vi "Create Command Packet 3.vi"(0 "CCD Format Parameters":T1={"Serial Origin"=50, "Serial Length"=512, "Serial Binning"=1, "Parallel Origin"=0, "Parallel Length"=1024, "Parallel Binning"=1} {"Parallel Binning" min=1 max=5000 step=1; "Parallel Length" min=0 max=65535 step=1; "Parallel Origin" min=0 max=9000 step=1; "Serial Binning" min=1 max=5000 step=1; "Serial Length" min=0 max=65535 step=1; "Serial Origin" min=0 max=9000 step=1}, 4 "Save As":u16(ring) items=["U16 FITS", "I16 FITS", "I32 FITS", "SGL FITS", "U16 TIFF", "I16 TIFF", "I32 TIFF", "SGL TIFF"], 5 "Acq. Mode/Type/Frame Mode/RO Mode":u8, 6 "File Name":string, 7 "Camera ID (1)":u8=1, 8 "Mode":u16, 9 "Exposure Time (ms)":u32, 10 "Buffer/Avg #/Frames":u16, 11 "Function #":u16) -> (2 "Cmd Packet":string)   [LabVIEW 2015]
uses:
  CCD Format.ctl
panel:
  # "Parallel"
  # "Serial"
  # "Origin"
  # "Length"
  # "Binning"
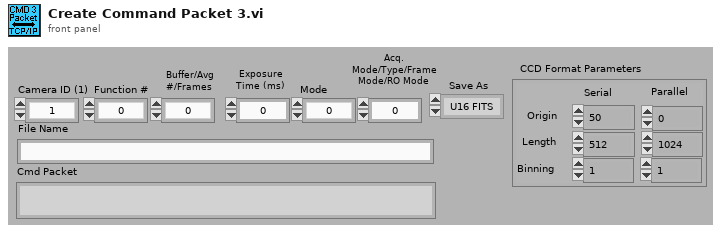
[diagram p1: front panel]
types:
  T1 = typedef "CCD Format.ctl" = cluster{"Serial Origin":i32, "Serial Length":i32, "Serial Binning":i32, "Parallel Origin":i32, "Parallel Length":i32, "Parallel Binning":i32}
  T2 = cluster{"Packet Length":u32, u8, "Camera ID (1)":u8, "Function #":u16, "Param Block Length":u16}
  T3 = cluster{u32, u8, "Camera ID (1)":u8, "Function #":u16, u16, "Exposure Time (ms)":u32, "Mode":u16, "Buffer/Avg #/Frames":u16, "Save As":u16}
  T4 = cluster{"Packet Length":u32, u8, "Camera ID (1)":u8, "Function #":u16, "Param Block Length":u16, "Buffer/Avg #/Frames":u16}
  T5 = cluster{u32, u8, "Camera ID (1)":u8, "Function #":u16, u16, "Buffer/Avg #/Frames":u16, "Save As":u16}
  T6 = cluster{"Packet Length":u32, u8, "Camera ID (1)":u8, "Function #":u16, "Param Block Length":u16, "Acq. Mode/Type/Frame Mode/RO Mode":u8}
  T7 = cluster{"Packet Length":u32, u8, "Camera ID (1)":u8, "Function #":u16, "Param Block Length":u16, "Exposure Time (ms)":u32}
  T8 = cluster{"Packet Length":u32, u8, "Camera ID (1)":u8, "Function #":u16, "Param Block Length":u16, "Buffer/Avg #/Frames":u16, "Acq. Mode/Type/Frame Mode/RO Mode":u8}
  T9 = cluster{u32, u8, "Camera ID (1)":u8, "Function #":u16, u16, "Mode":u16, "Buffer/Avg #/Frames":u16, "Save As":u16}
  T10 = cluster{"Packet Length":u32, u8, "Camera ID (1)":u8, "Function #":u16, "Param Block Length":u16, "CCD Format Parameters":T1}
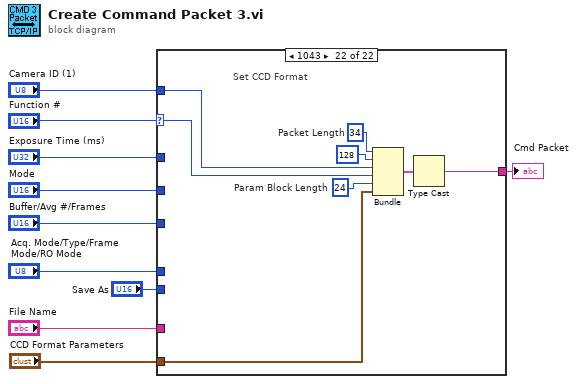
[diagram p0: block diagram]
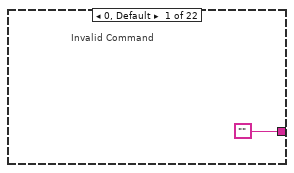
[diagram p2: hidden frame]
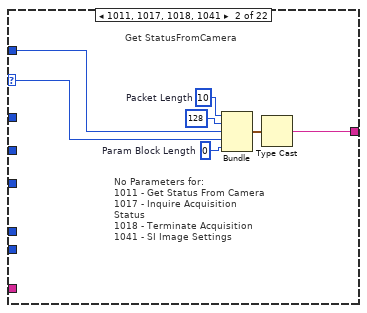
[diagram p3: hidden frame]
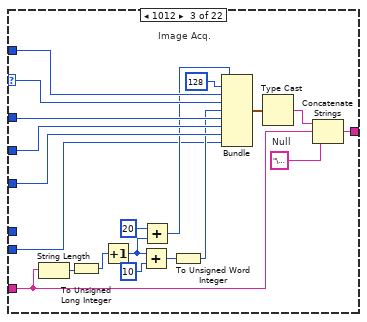
[diagram p4: hidden frame]
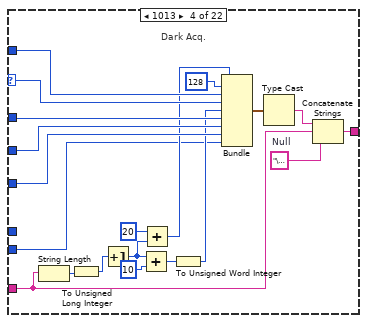
[diagram p5: hidden frame]
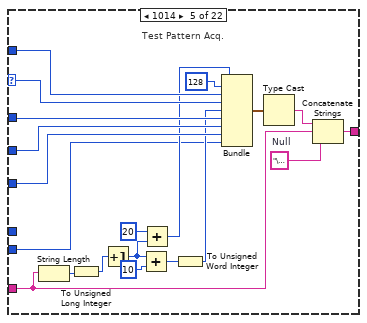
[diagram p6: hidden frame]
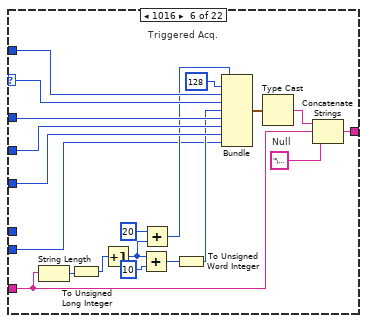
[diagram p7: hidden frame]
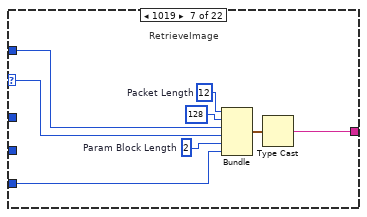
[diagram p8: hidden frame]
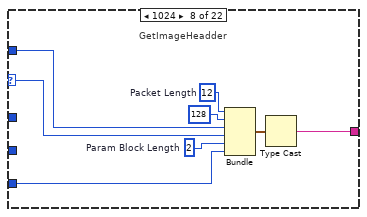
[diagram p9: hidden frame]
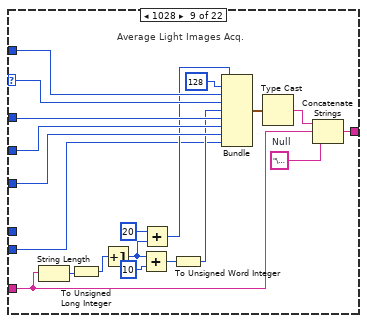
[diagram p10: hidden frame]
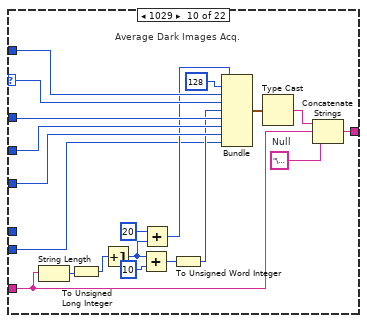
[diagram p11: hidden frame]
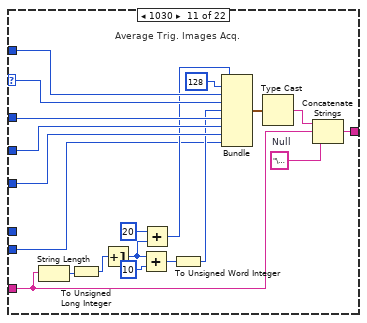
[diagram p12: hidden frame]
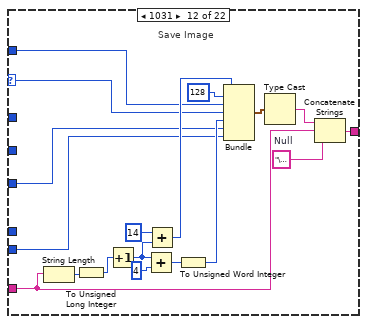
[diagram p13: hidden frame]
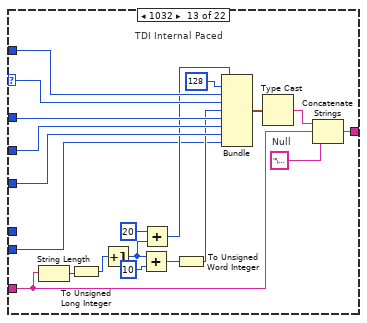
[diagram p14: hidden frame]
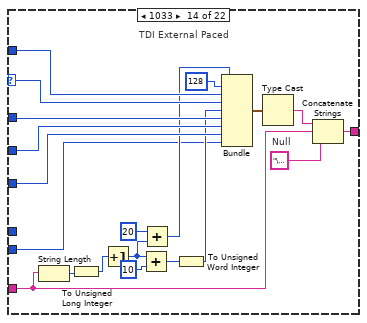
[diagram p15: hidden frame]
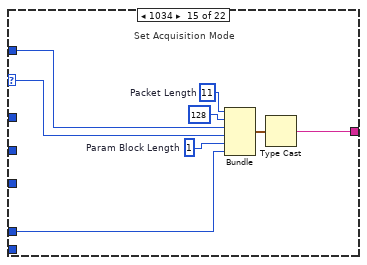
[diagram p16: hidden frame]
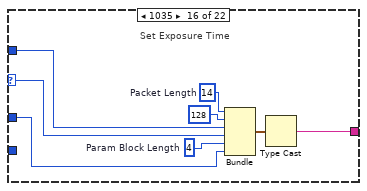
[diagram p17: hidden frame]
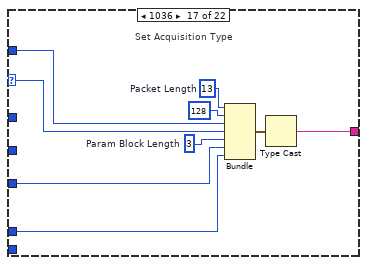
[diagram p18: hidden frame]
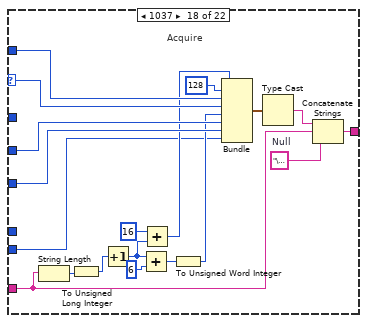
[diagram p19: hidden frame]
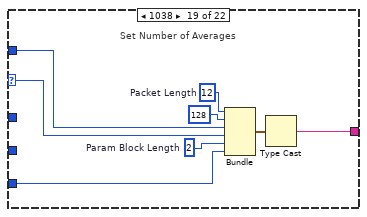
[diagram p20: hidden frame]
diagram:
  n1 = case shown="1043" "Function #" {
    selector: "Function #" -> [_ w15 w35 w55 w75 w95 w103 w109 w131 w151 w171 w176 w209 w229 w235 w243 w252 w273 w279 w287 w295 w303]
    tunnel: "Camera ID (1)" -> [_ w16 w36 w56 w76 w96 w104 w110 w132 w152 w172 w175 w210 w230 w236 w244 w253 w274 w280 w288 w296 w304]
    tunnel: "Exposure Time (ms)" -> [_ _ w34 w54 w74 w94 _ _ w130 w150 w170 _ w208 w228 _ w241 _ _ _ _ _ _]
    tunnel: "Mode" -> [_ _ w33 w53 w73 w93 _ _ w129 w149 w169 _ w207 w227 _ _ _ w272 _ _ _ _]
    tunnel: "Buffer/Avg #/Frames" -> [_ _ w32 w52 w72 w92 w102 w108 w128 w148 w168 w178 w206 w226 _ _ w249 w271 w277 w285 _ _]
    tunnel: "File Name" -> [_ _ w23 w43 w63 w83 _ _ w119 w139 w159 w180 w197 w217 _ _ _ w262 _ _ _ _]
    tunnel: ["" w12 w21 w41 w61 w81 w99 w107 w117 w137 w157 w177 w195 w215 w234 w242 w251 w260 w278 w286 w294 w302] -> w4
    tunnel: "Save As" -> [_ _ w19 w39 w59 w79 _ _ w115 w135 w155 w179 w193 w213 _ _ _ w258 _ _ _ _]
    tunnel: "Acq. Mode/Type/Frame Mode/RO Mode" -> [_ _ _ _ _ _ _ _ _ _ _ _ _ _ w233 _ w250 _ _ _ w293 _]
    tunnel: "CCD Format Parameters" -> [_ _ _ _ _ _ _ _ _ _ _ _ _ _ _ _ _ _ _ _ _ w301]
    frame 0, Default {
      # "Invalid Command"
    }
    frame 1011, 1017, 1018, 1041 {
      w13 = u16 0  # Param Block Length
      w14 = u32 10  # Packet Length
      # "No Parameters for:\n1011 - Get Status From Camera\n1017 - Inquire Acquisition Status\n1018 - Terminate Acquisition\n1041 - SI Image Settings"
      # "Get StatusFromCamera"
      n2 = Bundle("Packet Length"=w14, u8 128, "Camera ID (1)"=w16, "Function #"=w15, "Param Block Length"=w13) -> (w17:T2)  [unwired: 1 in]
      n3 = Type Cast(x=w17) -> (*(type *) &x=w12:string)  [unwired: 1 in]
    }
    frame 1012 {
      w22 = "\u0000"  # Null
      # "Image Acq."
      n4 = String Length(string=w23) -> (length=w31:i32)
      n5 = To Unsigned Long Integer(number=w31) -> (unsigned 32bit integer=w29:u32)
      n6 = Increment(x=w29) -> (x+1=w30:u32)
      n7 = Add(x=w30, y=u16 10) -> (x+y=w25:u32)
      n8 = Add(x=u16 20, y=w30) -> (x+y=w26:u32)
      n9 = To Unsigned Word Integer(number=w25) -> (unsigned 16bit integer=w20:u16)
      n10 = Bundle(w26, u8 128, "Camera ID (1)"=w36, "Function #"=w35, w20, "Exposure Time (ms)"=w34, "Mode"=w33, "Buffer/Avg #/Frames"=w32, "Save As"=w19) -> (w37:T3)  [unwired: 1 in]
      n11 = Type Cast(x=w37) -> (*(type *) &x=w24:string)  [unwired: 1 in]
      n12 = Concatenate Strings(w24, w23, w22) -> (w21:string)
    }
    frame 1013 {
      w42 = "\u0000"  # Null
      # "Dark Acq."
      n13 = String Length(string=w43) -> (length=w51:i32)
      n14 = To Unsigned Long Integer(number=w51) -> (unsigned 32bit integer=w49:u32)
      n15 = Increment(x=w49) -> (x+1=w50:u32)
      n16 = Add(x=w50, y=u16 10) -> (x+y=w45:u32)
      n17 = Add(x=u16 20, y=w50) -> (x+y=w46:u32)
      n18 = To Unsigned Word Integer(number=w45) -> (unsigned 16bit integer=w40:u16)
      n19 = Bundle(w46, u8 128, "Camera ID (1)"=w56, "Function #"=w55, w40, "Exposure Time (ms)"=w54, "Mode"=w53, "Buffer/Avg #/Frames"=w52, "Save As"=w39) -> (w57:T3)  [unwired: 1 in]
      n20 = Type Cast(x=w57) -> (*(type *) &x=w44:string)  [unwired: 1 in]
      n21 = Concatenate Strings(w44, w43, w42) -> (w41:string)
    }
    frame 1014 {
      w62 = "\u0000"  # Null
      # "Test Pattern Acq."
      n22 = String Length(string=w63) -> (length=w71:i32)
      n23 = To Unsigned Long Integer(number=w71) -> (unsigned 32bit integer=w69:u32)
      n24 = Increment(x=w69) -> (x+1=w70:u32)
      n25 = Add(x=w70, y=u16 10) -> (x+y=w65:u32)
      n26 = Add(x=u16 20, y=w70) -> (x+y=w66:u32)
      n27 = To Unsigned Word Integer(number=w65) -> (unsigned 16bit integer=w60:u16)
      n28 = Bundle(w66, u8 128, "Camera ID (1)"=w76, "Function #"=w75, w60, "Exposure Time (ms)"=w74, "Mode"=w73, "Buffer/Avg #/Frames"=w72, "Save As"=w59) -> (w77:T3)  [unwired: 1 in]
      n29 = Type Cast(x=w77) -> (*(type *) &x=w64:string)  [unwired: 1 in]
      n30 = Concatenate Strings(w64, w63, w62) -> (w61:string)
    }
    frame 1016 {
      w82 = "\u0000"  # Null
      # "Triggered Acq."
      n31 = String Length(string=w83) -> (length=w91:i32)
      n32 = To Unsigned Long Integer(number=w91) -> (unsigned 32bit integer=w89:u32)
      n33 = Increment(x=w89) -> (x+1=w90:u32)
      n34 = Add(x=w90, y=u16 10) -> (x+y=w85:u32)
      n35 = Add(x=u16 20, y=w90) -> (x+y=w86:u32)
      n36 = To Unsigned Word Integer(number=w85) -> (unsigned 16bit integer=w80:u16)
      n37 = Bundle(w86, u8 128, "Camera ID (1)"=w96, "Function #"=w95, w80, "Exposure Time (ms)"=w94, "Mode"=w93, "Buffer/Avg #/Frames"=w92, "Save As"=w79) -> (w97:T3)  [unwired: 1 in]
      n38 = Type Cast(x=w97) -> (*(type *) &x=w84:string)  [unwired: 1 in]
      n39 = Concatenate Strings(w84, w83, w82) -> (w81:string)
    }
    frame 1019 {
      w100 = u16 2  # Param Block Length
      w101 = u32 12  # Packet Length
      # "RetrieveImage"
      n40 = Bundle("Packet Length"=w101, u8 128, "Camera ID (1)"=w104, "Function #"=w103, "Param Block Length"=w100, "Buffer/Avg #/Frames"=w102) -> (w105:T4)  [unwired: 1 in]
      n41 = Type Cast(x=w105) -> (*(type *) &x=w99:string)  [unwired: 1 in]
    }
    frame 1024 {
      w111 = u16 2  # Param Block Length
      w112 = u32 12  # Packet Length
      # "GetImageHeadder"
      n42 = Bundle("Packet Length"=w112, u8 128, "Camera ID (1)"=w110, "Function #"=w109, "Param Block Length"=w111, "Buffer/Avg #/Frames"=w108) -> (w113:T4)  [unwired: 1 in]
      n43 = Type Cast(x=w113) -> (*(type *) &x=w107:string)  [unwired: 1 in]
    }
    frame 1028 {
      w118 = "\u0000"  # Null
      # "Average Light Images Acq."
      n44 = String Length(string=w119) -> (length=w127:i32)
      n45 = To Unsigned Long Integer(number=w127) -> (unsigned 32bit integer=w125:u32)
      n46 = Increment(x=w125) -> (x+1=w126:u32)
      n47 = Add(x=w126, y=u16 10) -> (x+y=w121:u32)
      n48 = Add(x=u16 20, y=w126) -> (x+y=w122:u32)
      n49 = To Unsigned Word Integer(number=w121) -> (unsigned 16bit integer=w116:u16)
      n50 = Bundle(w122, u8 128, "Camera ID (1)"=w132, "Function #"=w131, w116, "Exposure Time (ms)"=w130, "Mode"=w129, "Buffer/Avg #/Frames"=w128, "Save As"=w115) -> (w133:T3)  [unwired: 1 in]
      n51 = Type Cast(x=w133) -> (*(type *) &x=w120:string)  [unwired: 1 in]
      n52 = Concatenate Strings(w120, w119, w118) -> (w117:string)
    }
    frame 1029 {
      w138 = "\u0000"  # Null
      # "Average Dark Images Acq."
      n53 = String Length(string=w139) -> (length=w147:i32)
      n54 = To Unsigned Long Integer(number=w147) -> (unsigned 32bit integer=w145:u32)
      n55 = Increment(x=w145) -> (x+1=w146:u32)
      n56 = Add(x=w146, y=u16 10) -> (x+y=w141:u32)
      n57 = Add(x=u16 20, y=w146) -> (x+y=w142:u32)
      n58 = To Unsigned Word Integer(number=w141) -> (unsigned 16bit integer=w136:u16)
      n59 = Bundle(w142, u8 128, "Camera ID (1)"=w152, "Function #"=w151, w136, "Exposure Time (ms)"=w150, "Mode"=w149, "Buffer/Avg #/Frames"=w148, "Save As"=w135) -> (w153:T3)  [unwired: 1 in]
      n60 = Type Cast(x=w153) -> (*(type *) &x=w140:string)  [unwired: 1 in]
      n61 = Concatenate Strings(w140, w139, w138) -> (w137:string)
    }
    frame 1030 {
      w158 = "\u0000"  # Null
      # "Average Trig. Images Acq."
      n62 = String Length(string=w159) -> (length=w167:i32)
      n63 = To Unsigned Long Integer(number=w167) -> (unsigned 32bit integer=w165:u32)
      n64 = Increment(x=w165) -> (x+1=w166:u32)
      n65 = Add(x=w166, y=u16 10) -> (x+y=w161:u32)
      n66 = Add(x=u16 20, y=w166) -> (x+y=w162:u32)
      n67 = To Unsigned Word Integer(number=w161) -> (unsigned 16bit integer=w156:u16)
      n68 = Bundle(w162, u8 128, "Camera ID (1)"=w172, "Function #"=w171, w156, "Exposure Time (ms)"=w170, "Mode"=w169, "Buffer/Avg #/Frames"=w168, "Save As"=w155) -> (w173:T3)  [unwired: 1 in]
      n69 = Type Cast(x=w173) -> (*(type *) &x=w160:string)  [unwired: 1 in]
      n70 = Concatenate Strings(w160, w159, w158) -> (w157:string)
    }
    frame 1031 {
      w182 = "\u0000"  # Null
      # "Save Image"
      n71 = String Length(string=w180) -> (length=w190:i32)
      n72 = To Unsigned Long Integer(number=w190) -> (unsigned 32bit integer=w188:u32)
      n73 = Increment(x=w188) -> (x+1=w189:u32)
      n74 = Add(x=w189, y=u16 4) -> (x+y=w184:u32)
      n75 = Add(x=u16 14, y=w189) -> (x+y=w185:u32)
      n76 = To Unsigned Word Integer(number=w184) -> (unsigned 16bit integer=w181:u16)
      n77 = Bundle(w185, u8 128, "Camera ID (1)"=w175, "Function #"=w176, w181, "Buffer/Avg #/Frames"=w178, "Save As"=w179) -> (w191:T5)  [unwired: 1 in]
      n78 = Type Cast(x=w191) -> (*(type *) &x=w183:string)  [unwired: 1 in]
      n79 = Concatenate Strings(w183, w180, w182) -> (w177:string)
    }
    frame 1032 {
      w196 = "\u0000"  # Null
      # "TDI Internal Paced"
      n80 = String Length(string=w197) -> (length=w205:i32)
      n81 = To Unsigned Long Integer(number=w205) -> (unsigned 32bit integer=w203:u32)
      n82 = Increment(x=w203) -> (x+1=w204:u32)
      n83 = Add(x=w204, y=u16 10) -> (x+y=w199:u32)
      n84 = Add(x=u16 20, y=w204) -> (x+y=w200:u32)
      n85 = To Unsigned Word Integer(number=w199) -> (unsigned 16bit integer=w194:u16)
      n86 = Bundle(w200, u8 128, "Camera ID (1)"=w210, "Function #"=w209, w194, "Exposure Time (ms)"=w208, "Mode"=w207, "Buffer/Avg #/Frames"=w206, "Save As"=w193) -> (w211:T3)  [unwired: 1 in]
      n87 = Type Cast(x=w211) -> (*(type *) &x=w198:string)  [unwired: 1 in]
      n88 = Concatenate Strings(w198, w197, w196) -> (w195:string)
    }
    frame 1033 {
      w216 = "\u0000"  # Null
      # "TDI External Paced"
      n89 = String Length(string=w217) -> (length=w225:i32)
      n90 = To Unsigned Long Integer(number=w225) -> (unsigned 32bit integer=w223:u32)
      n91 = Increment(x=w223) -> (x+1=w224:u32)
      n92 = Add(x=w224, y=u16 10) -> (x+y=w219:u32)
      n93 = Add(x=u16 20, y=w224) -> (x+y=w220:u32)
      n94 = To Unsigned Word Integer(number=w219) -> (unsigned 16bit integer=w214:u16)
      n95 = Bundle(w220, u8 128, "Camera ID (1)"=w230, "Function #"=w229, w214, "Exposure Time (ms)"=w228, "Mode"=w227, "Buffer/Avg #/Frames"=w226, "Save As"=w213) -> (w231:T3)  [unwired: 1 in]
      n96 = Type Cast(x=w231) -> (*(type *) &x=w218:string)  [unwired: 1 in]
      n97 = Concatenate Strings(w218, w217, w216) -> (w215:string)
    }
    frame 1034 {
      w237 = u16 1  # Param Block Length
      w238 = u32 11  # Packet Length
      # "Set Acquisition Mode"
      n98 = Bundle("Packet Length"=w238, u8 128, "Camera ID (1)"=w236, "Function #"=w235, "Param Block Length"=w237, "Acq. Mode/Type/Frame Mode/RO Mode"=w233) -> (w239:T6)  [unwired: 1 in]
      n99 = Type Cast(x=w239) -> (*(type *) &x=w234:string)  [unwired: 1 in]
    }
    frame 1035 {
      w245 = u16 4  # Param Block Length
      w246 = u32 14  # Packet Length
      # "Set Exposure Time"
      n100 = Bundle("Packet Length"=w246, u8 128, "Camera ID (1)"=w244, "Function #"=w243, "Param Block Length"=w245, "Exposure Time (ms)"=w241) -> (w247:T7)  [unwired: 1 in]
      n101 = Type Cast(x=w247) -> (*(type *) &x=w242:string)  [unwired: 1 in]
    }
    frame 1036 {
      w254 = u16 3  # Param Block Length
      w255 = u32 13  # Packet Length
      # "Set Acquisition Type"
      n102 = Bundle("Packet Length"=w255, u8 128, "Camera ID (1)"=w253, "Function #"=w252, "Param Block Length"=w254, "Buffer/Avg #/Frames"=w249, "Acq. Mode/Type/Frame Mode/RO Mode"=w250) -> (w256:T8)  [unwired: 1 in]
      n103 = Type Cast(x=w256) -> (*(type *) &x=w251:string)  [unwired: 1 in]
    }
    frame 1037 {
      w261 = "\u0000"  # Null
      # "Acquire"
      n104 = String Length(string=w262) -> (length=w270:i32)
      n105 = To Unsigned Long Integer(number=w270) -> (unsigned 32bit integer=w268:u32)
      n106 = Increment(x=w268) -> (x+1=w269:u32)
      n107 = Add(x=w269, y=u16 6) -> (x+y=w264:u32)
      n108 = Add(x=u16 16, y=w269) -> (x+y=w265:u32)
      n109 = To Unsigned Word Integer(number=w264) -> (unsigned 16bit integer=w259:u16)
      n110 = Bundle(w265, u8 128, "Camera ID (1)"=w274, "Function #"=w273, w259, "Mode"=w272, "Buffer/Avg #/Frames"=w271, "Save As"=w258) -> (w275:T9)  [unwired: 1 in]
      n111 = Type Cast(x=w275) -> (*(type *) &x=w263:string)  [unwired: 1 in]
      n112 = Concatenate Strings(w263, w262, w261) -> (w260:string)
    }
    frame 1038 {
      w281 = u16 2  # Param Block Length
      w282 = u32 12  # Packet Length
      # "Set Number of Averages"
      n113 = Bundle("Packet Length"=w282, u8 128, "Camera ID (1)"=w280, "Function #"=w279, "Param Block Length"=w281, "Buffer/Avg #/Frames"=w277) -> (w283:T4)  [unwired: 1 in]
      n114 = Type Cast(x=w283) -> (*(type *) &x=w278:string)  [unwired: 1 in]
    }
    frame 1039 {
      w289 = u16 2  # Param Block Length
      w290 = u32 12  # Packet Length
      # "Set Number of Frames"
      n115 = Bundle("Packet Length"=w290, u8 128, "Camera ID (1)"=w288, "Function #"=w287, "Param Block Length"=w289, "Buffer/Avg #/Frames"=w285) -> (w291:T4)  [unwired: 1 in]
      n116 = Type Cast(x=w291) -> (*(type *) &x=w286:string)  [unwired: 1 in]
    }
    frame 1040, 1042 {
      w297 = u16 1  # Param Block Length
      w298 = u32 11  # Packet Length
      # "Set Multi-Frame Acquisition Buffer Mode\nor Set RO Mode"
      n117 = Bundle("Packet Length"=w298, u8 128, "Camera ID (1)"=w296, "Function #"=w295, "Param Block Length"=w297, "Acq. Mode/Type/Frame Mode/RO Mode"=w293) -> (w299:T6)  [unwired: 1 in]
      n118 = Type Cast(x=w299) -> (*(type *) &x=w294:string)  [unwired: 1 in]
    }
    frame 1043 {
      w305 = u16 24  # Param Block Length
      w306 = u32 34  # Packet Length
      # "Set CCD Format"
      n119 = Bundle("Packet Length"=w306, u8 128, "Camera ID (1)"=w304, "Function #"=w303, "Param Block Length"=w305, "CCD Format Parameters"=w301) -> (w307:T10)  [unwired: 1 in]
      n120 = Type Cast(x=w307) -> (*(type *) &x=w302:string)  [unwired: 1 in]
    }
  }
  "Cmd Packet" <- w4
